vi "PM100D_Zeroing.vi"(5 "VISA In":refnum<visa-resource-name>) -> (1 "ZeroValue":dbl)   [LabVIEW 2009]
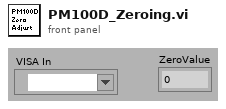
[diagram p1: front panel]
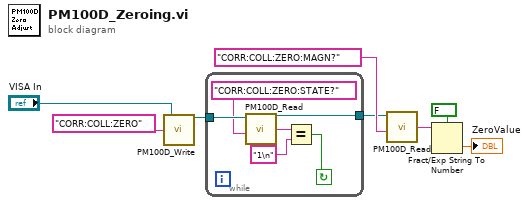
[diagram p0: block diagram]
diagram:
  n1 = call "PM100D_Write.vi"("Command"="CORR:COLL:ZERO", "VISA in"="VISA In") -> ("VISA out"=w6:refnum<visa-resource-name>)  [unwired: 1 in, 1 out]
  n2 = while {
    tunnel: w6 -> [w14]
    tunnel: [w9] -> w7
    stop <- w10 continue-if-true
    n3 = call "PM100D_Read.vi"("Command"="CORR:COLL:ZERO:STATE?", "VISA in"=w14) -> ("ReadValue"=w12:string, "VISA out"=w9:refnum<visa-resource-name>)  [unwired: 2 in, 1 out]
    n4 = Equal?(x=w12, y="1\n") -> (x = y?=w10:bool)
  }
  n5 = call "PM100D_Read.vi"("Command"="CORR:COLL:ZERO:MAGN?", "VISA in"=w7) -> ("ReadValue"=w3:string)  [unwired: 2 in, 2 out]
  n6 = Fract/Exp String To Number(use system decimal point (T)=FALSE, string=w3) -> (number=→"ZeroValue":dbl)  [unwired: 2 in, 1 out]
